vi "AddNode.vi"(8 "error in":errorcluster, 9 "node in":refnum<class "NISE_CEF_Node.lvclass">, 10 "parent node ID":string) -> (0 "error out":errorcluster, 2 "summary":T1[](array[typedef]))   [LabVIEW 2013, in "NISE_CEF_TreeControl.lvlib"]
doc: "This Vi adds a new node to the Parent Node ID"
uses:
  NISE_CEF_TreeControl.lvlib
  Node/Summary.ctl
  Node/NISE_CEF_Node.lvclass
  Node/NISE_CEF_Node.lvclass/NISE_CEF_Node.ctl
  Node/ReadChildren.vi
  Node/WriteParent.vi
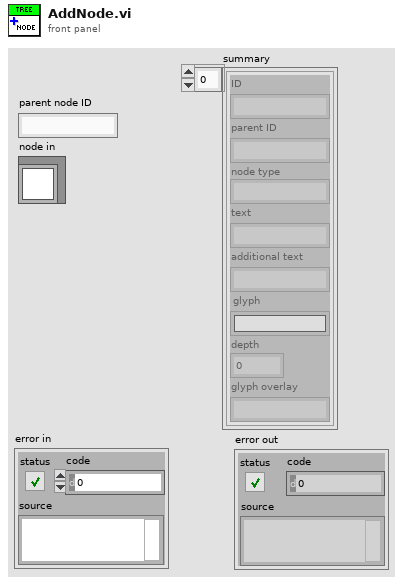
[diagram p1: front panel]
types:
  T1 = typedef "NISE_CEF_Node.lvclass/Summary.ctl" = cluster{"ID":string, "parent ID":string, "node type":string, "text":string, "additional text":string, "glyph":string, "depth":i32, "glyph overlay":string}
  T2 = typedef "NISE_CEF_Node.lvclass/NodeRef.ctl" = refnum<data-value>
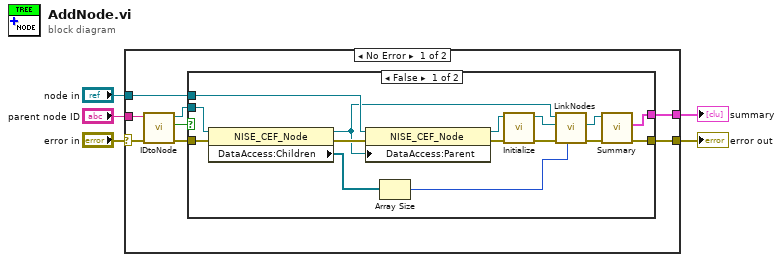
[diagram p0: block diagram]
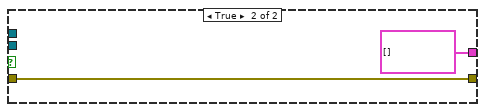
[diagram p2: hidden frame]
diagram:
  n1 = case shown="No Error" "error in" {
    selector: "error in" -> [w8 w31]
    tunnel: "parent node ID" -> [w13 _]
    tunnel: [w11 _] -> w3
    tunnel: [w10 w31] -> w2
    tunnel: "node in" -> [w9 _]
    frame No Error {
      n2 = call "IDtoNode.vi"("error in"=w8, "ID"=w13) -> ("error out"=w7:errorcluster, "invalid Id"=w6:bool, "node ref"=w12:T2)  [unwired: 7 in]
      n3 = case shown="False" w6 {
        tunnel: w12 -> [w22 _]
        tunnel: [w28 T1[] [] ("summary")] -> w11
        tunnel: [w27 w30] -> w10
        tunnel: w9 -> [w16 _]
        tunnel: w7 -> [w19 w30]
        frame False {
          n4 = property class="NISE_CEF_Node"(reference=w22, error in=w19) -> (reference out=w14:T2, error out=w18:errorcluster, "DataAccess:Children"=w21:T2[])
          n5 = property class="NISE_CEF_Node"(reference=w16, error in=w18, "DataAccess:Parent"=w14) -> (reference out=w15:refnum<class "NISE_CEF_Node.lvclass">, error out=w17:errorcluster)
          n6 = Array Size(array=w21) -> (size(s)=w20:i32)
          n7 = call-dynamic "Initialize.vi"("error in"=w17, "node in"=w15) -> ("error out"=w23:errorcluster, "data value reference"=w24:T2)  [unwired: 7 in, 1 out]
          n8 = call "LinkNodes.vi"("index"=w20, "error in"=w23, "child in"=w24, "parent in"=w14) -> ("error out"=w26:errorcluster, "child out"=w25:T2)  [unwired: 5 in, 1 out]
          n9 = call "Summary.vi"("error in"=w26, "node self ref"=w25) -> ("error out"=w27:errorcluster, "summary"=w28:T1[])  [unwired: 8 in]
        }
        frame True {
        }
      }
    }
    frame Error {
    }
  }
  "error out" <- w2
  "summary" <- w3
